vi "init.vi"(8 "error in (no error)":errorcluster, 10 "Variant":variant, 11 "USB IO in":refnum<class "USB IO.lvclass">) -> (0 "error out":errorcluster, 3 "USB IO out":refnum<class "USB IO.lvclass">)   [LabVIEW 2025, in "USB IO.lvlib" / "USB IO.lvclass"]
uses:
  USB IO.lvclass
  USB IO.lvclass/USB IO.ctl
  <vilib>/DAQmx/create/channels.llb/DAQmx Create Channel (DO-Digital Output).vi
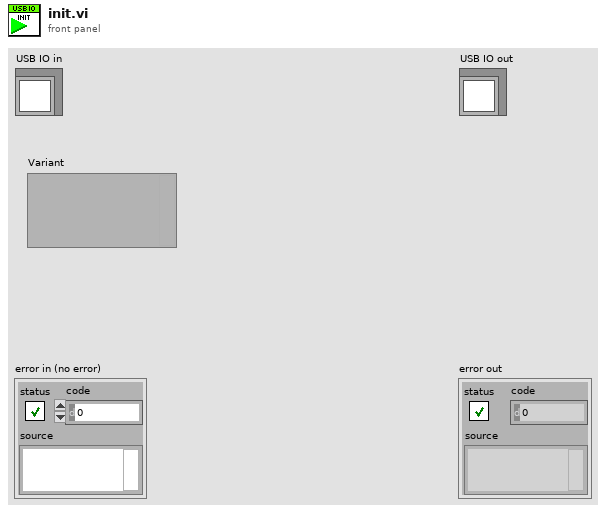
[diagram p1: front panel]
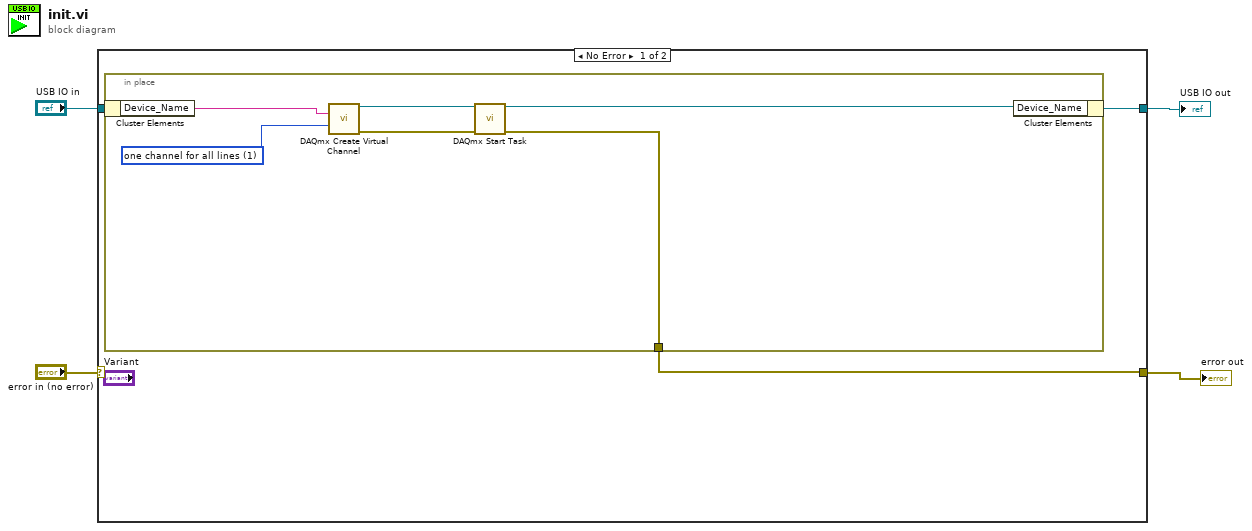
[diagram p0: block diagram]
diagram:
  n1 = case shown="No Error" "error in (no error)" {
    selector: "error in (no error)" -> [_ w15]
    tunnel: [w5 w15] -> w3
    tunnel: [w6 w14] -> w1
    tunnel: "USB IO in" -> [w7 w14]
    frame No Error {
      n2 = in-place {
        in-place-border: [w8] -> w5
        w12 = 1 items=["one channel for each line", "one channel for all lines"] ("line grouping")
        n3 = in-place-cluster #1(w7) -> ("Device_Name"=w13:string)
        n4 = call-poly <vilib>:"DAQmx Create Virtual Channel.vi"("lines"=w13, "line grouping"=w12) -> ("task out"=w11:refnum<k21>, "error out"=w10:errorcluster)  [unwired: 12 in]
        n5 = call <vilib>:"DAQmx Start Task.vi"("task/channels in"=w11, "error in"=w10) -> ("task out"=w9:refnum<k21>, "error out"=w8:errorcluster)  [unwired: 12 in]
        n6 = in-place-cluster #1("Device_Name"=w9) -> (w6:refnum<class "USB IO.lvclass">)
      }
    }
    frame Error {
    }
  }
  "error out" <- w3
  "USB IO out" <- w1
